vi "Get Sub-VI List with Levels for VI List.vi"(0 "VI List":string[](array[string]), 5 "Level (0)":i32, 9 "Recursive (T)":bool=TRUE, 11 "error in (no error)":errorcluster) -> (4 "VI Path List":path[](array[path]), 6 "VI Paths":path[](array[path]), 8 "VI Levels":i32[](array[numeric]), 15 "error out":errorcluster)   [LabVIEW 2010]
doc: "<B>Name:</B>\nBT - Get Sub-VI List with Levels for VI List.vi\n<B>References:</B>\nN/A\n<B>Function Description:</B>\nThis VI lists sub-VI paths and the associated hierarchy levels of the sub-VIs for the VIs specified by VI List. The paths of the input VI Names are returned at VI Path List. This VI uses recursion to evaluate the VI hierarchies of the VI List.\n\n<B>Inputs:</B>\nVI List: This is an array of VI names that will have all sub-VI paths returned at Sub-VI Paths.\n\nLevel (0): This is the hierarchy level of the VIs specified by VI List. Level 0 indicates that the VI is a top-level VI. Level 1 indicates a sub-VI that is contained on a top-level VI diagram. All VIs in the VI List are treated as being at this Level.\n\nRecursive (T): This Boolean is normally TRUE. When TRUE all sub-VI hierarchy levels will be listed. When FALSE, only the first level sub-VIs of the VI specified by VI Name will be listed.\n\nerror in (no error): Standard error in cluster\n\n<B>Outputs:</B>\nVI Path List: This is the array of paths for the VIs specified by VI List.\n\nSub-VI Paths: This is a list of paths for the sub-VIs of the VIs specified by VI List. When Recursive is TRUE, all sub-VI levels are included. When Recursive is FALSE, only first level sub-VIs of the VIs specified by VI List are listed.\n\nSub-VI Levels: This array has the same number of elements as and correlates with the Sub-VI Paths array. An element value of 1 indicates that the corresponding sub-VI is a first-level sub-VI and a value of 2 indicates that the corresponding sub-VI is a second-level sub-VI. The levels returned are relative to the level of the VI specified by VI Name and Level inputs.\n\nerror out: Standard error out cluster\n\n<B>Globals:</B>\nN/A\n<B>TestStand Variables:</B>\nN/A\n<B>User Guide:</B>\nN/A\n<B>Control Usage Rules:</B>\nN/A\n<B>VI Interaction:</B>\nN/A\n<B>Occurences:</B>\nN/A\n<B>Devices:</B>\nN/A\n<B>Files:</B>\nN/A\n<B>System Calls:</B>\nN/A\n<B>Keywords:</B>\ntools\n\nAuthor: spcase\nCurrent Revision: 48\nVSS Version: 1\nCopyright 2002 VI Engineering, Inc."
panel:
  in  "Get Callees Refnum":refnum<vi>
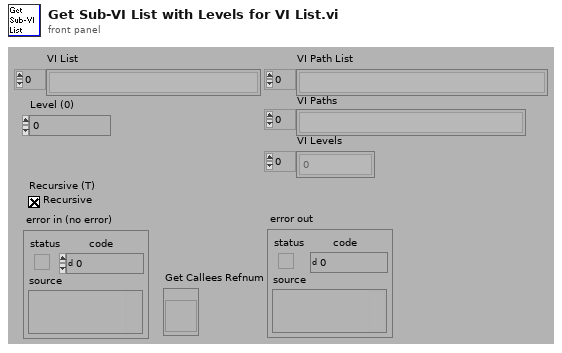
[diagram p1: front panel]
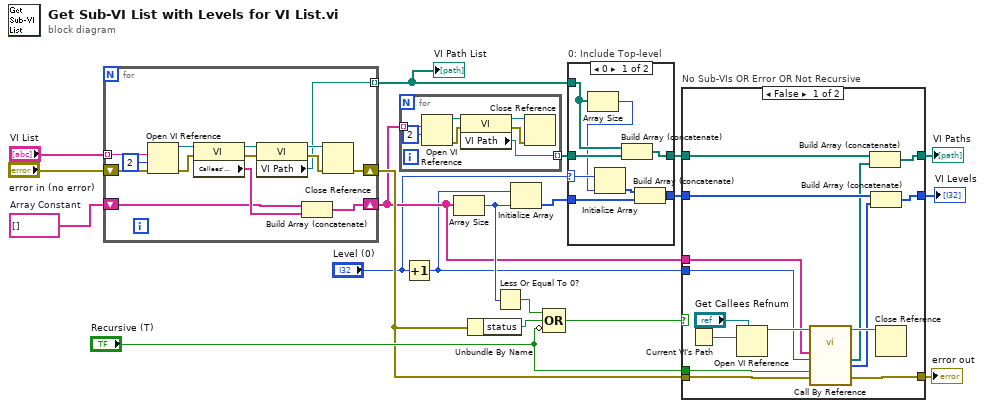
[diagram p0: block diagram]
diagram:
  w9 = string[] []  # Array Constant
  n1 = for {
    tunnel: [w28] -> w3 mode=indexing
    tunnel: "VI List" -> [w27] mode=indexing
    shift-right: [w25] -> w10
    shift-left: "error in (no error)" -> [w26]
    shift-right: [w22] -> w8
    shift-left: w9 -> [w21]
    n2 = Open VI Reference(vi path=w27, options=2, error in (no error)=w26) -> (vi reference=w33:refnum<vi>, error out=w34:errorcluster)  [unwired: 3 in]
    n3 = property class="VI"(reference=w33, error in=w34) -> (reference out=w31:refnum<vi>, error out=w30:errorcluster, "Callees' Names"=w23:string[])
    n4 = property class="VI"(reference=w31, error in=w30) -> (reference out=w32:refnum<vi>, error out=w29:errorcluster, "VI Path"=w28:path)
    n5 = Build Array (concatenate)(w21, w23) -> (w22:string[])
    n6 = Close Reference(reference=w32, error in (no error)=w29) -> (error out=w25:errorcluster)
  }
  "VI Path List" <- w3
  n7 = for {
    tunnel: w8 -> [w41] mode=indexing
    tunnel: [w36] -> w6 mode=indexing
    n8 = Open VI Reference(vi path=w41, options=2) -> (vi reference=w40:refnum<vi>, error out=w39:errorcluster)  [unwired: 4 in]
    n9 = property class="VI"(reference=w40, error in=w39) -> (reference out=w38:refnum<vi>, error out=w37:errorcluster, "VI Path"=w36:path)
    n10 = Close Reference(reference=w38, error in (no error)=w37) -> ()  [unwired: 1 out]
  }
  n11 = Increment(x="Level (0)") -> (x+1=w2:i32)
  n12 = Array Size(array=w8) -> (size(s)=w18:i32)
  n13 = Unbundle By Name(w10) -> ("status"=w16:bool)
  n14 = Less Or Equal To 0?(x=w18) -> (x <= 0?=w17:bool)
  n15 = Initialize Array(w2, w18) -> (w7:i32[])
  n16 = Compound Arithmetic op=OR(w17, w16, invert "Recursive (T)") -> (w15:bool)
  n17 = case "0: Include Top-level" shown="0" "Level (0)" {
    selector: "Level (0)" -> [w45 _]
    tunnel: w6 -> [w47 w51]
    tunnel: w7 -> [w49 w50]
    tunnel: [w46 w51] -> w5
    tunnel: [w48 w50] -> w4
    tunnel: w3 -> [w43 _]
    frame 0 {
      n18 = Array Size(array=w43) -> (size(s)=w42:i32)
      n19 = Initialize Array(w45, w42) -> (w44:i32[])
      n20 = Build Array (concatenate)(w43, w47) -> (w46:path[])
      n21 = Build Array (concatenate)(w44, w49) -> (w48:i32[])
    }
    frame 1, Default {
    }
  }
  n22 = case "No Sub-VIs OR Error OR Not Recursive" shown="False" w15 {
    tunnel: w4 -> [w56 w69]
    tunnel: [w62 w67] -> w13
    tunnel: [w61 w69] -> w20
    tunnel: w10 -> [w60 w68]
    tunnel: [w59 w68] -> w19
    tunnel: "Recursive (T)" -> [w58 _]
    tunnel: w5 -> [w55 w67]
    tunnel: w2 -> [w57 _]
    tunnel: w8 -> [w54 _]
    frame False {
      n23 = Current VI's Path() -> (path=w65:path)
      n24 = Open VI Reference(type specifier VI Refnum (for type only)="Get Callees Refnum", vi path=w65) -> (vi reference=w64:refnum<vi>)  [unwired: 4 in, 1 out]
      n25 = call-by-ref "?"(reference=w64, "VI List"=w54, "Level (0)"=w57, "Recursive (T)"=w58, "error in (no error)"=w60) -> (reference out=w63:refnum<vi>, "Sub-VI Paths"=w52:path[], "Sub-VI Levels"=w53:i32[], "error out"=w59:errorcluster)  [unwired: 9 in, 2 out]
      n26 = Build Array (concatenate)(w55, w52) -> (w62:path[])
      n27 = Build Array (concatenate)(w56, w53) -> (w61:i32[])
      n28 = Close Reference(reference=w63) -> ()  [unwired: 1 in, 1 out]
    }
    frame True {
    }
  }
  "error out" <- w19
  "VI Paths" <- w13
  "VI Levels" <- w20
